vi "ROI_Setting_UI.vi"(8 "error in (no error)":errorcluster, 11 "Vision_Image":T1(plugin-control)) -> (0 "error out":errorcluster)   [LabVIEW 2019]
uses:
  Controls/ROI_List_Action.ctl
panel:
  in  "Exit":bool
  in  "RemoveROI":bool
  in  "CreateROI":bool
  in  "ROI List":i32[](listbox)
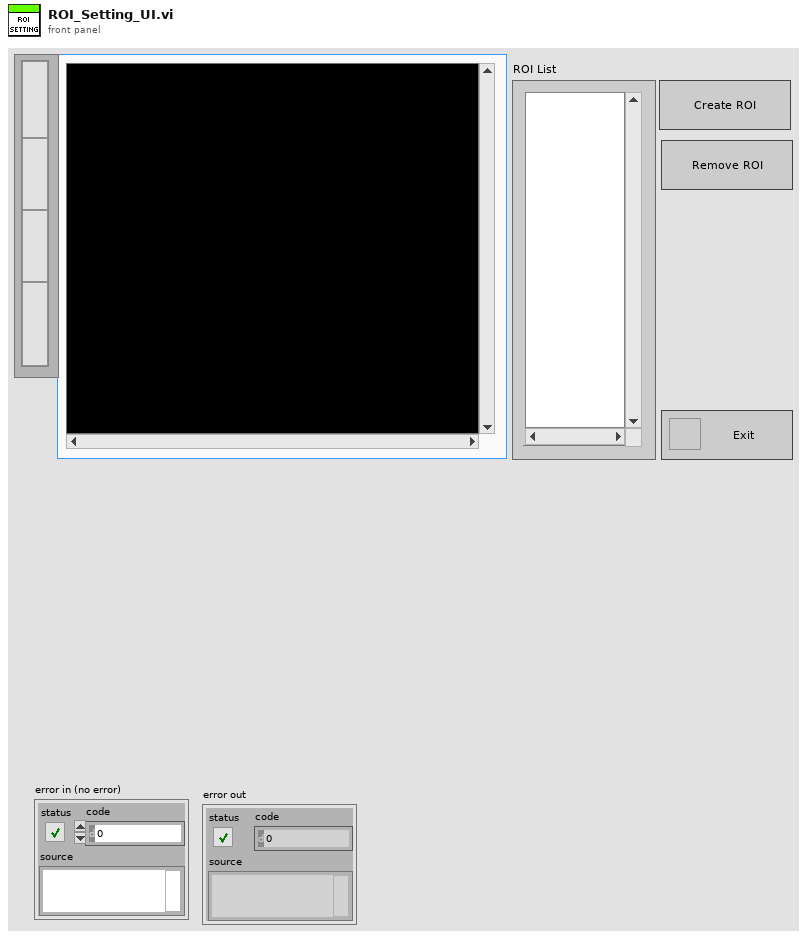
[diagram p1: front panel]
types:
  T1 = typedef "IMAQ Image.ctl" = refnum<image>
  T2 = typedef "ROI_List_Action.ctl" = enum16{"Init", "Add ROI", "Delete ROI", "Get All ROI", "Get Specific ROI", "Set Analysis Setting", "Set Process Setting", "Replace All Entries", "ROIEntryBackup", "ROIEntryBackupClear", "ROIEntryReturn"}
  T3 = cluster{"Global Rectangle":i32[], "Contours":cluster{"Contour Type":u32, "ROI Type":u32, "Points":i32[]}[]}
  T4 = cluster{"Contour Type":u32, "ROI Type":u32, "Points":i32[]}[]
  T5 = cluster{"Contour Type":u32, "ROI Type":u32, "Points":i32[]}
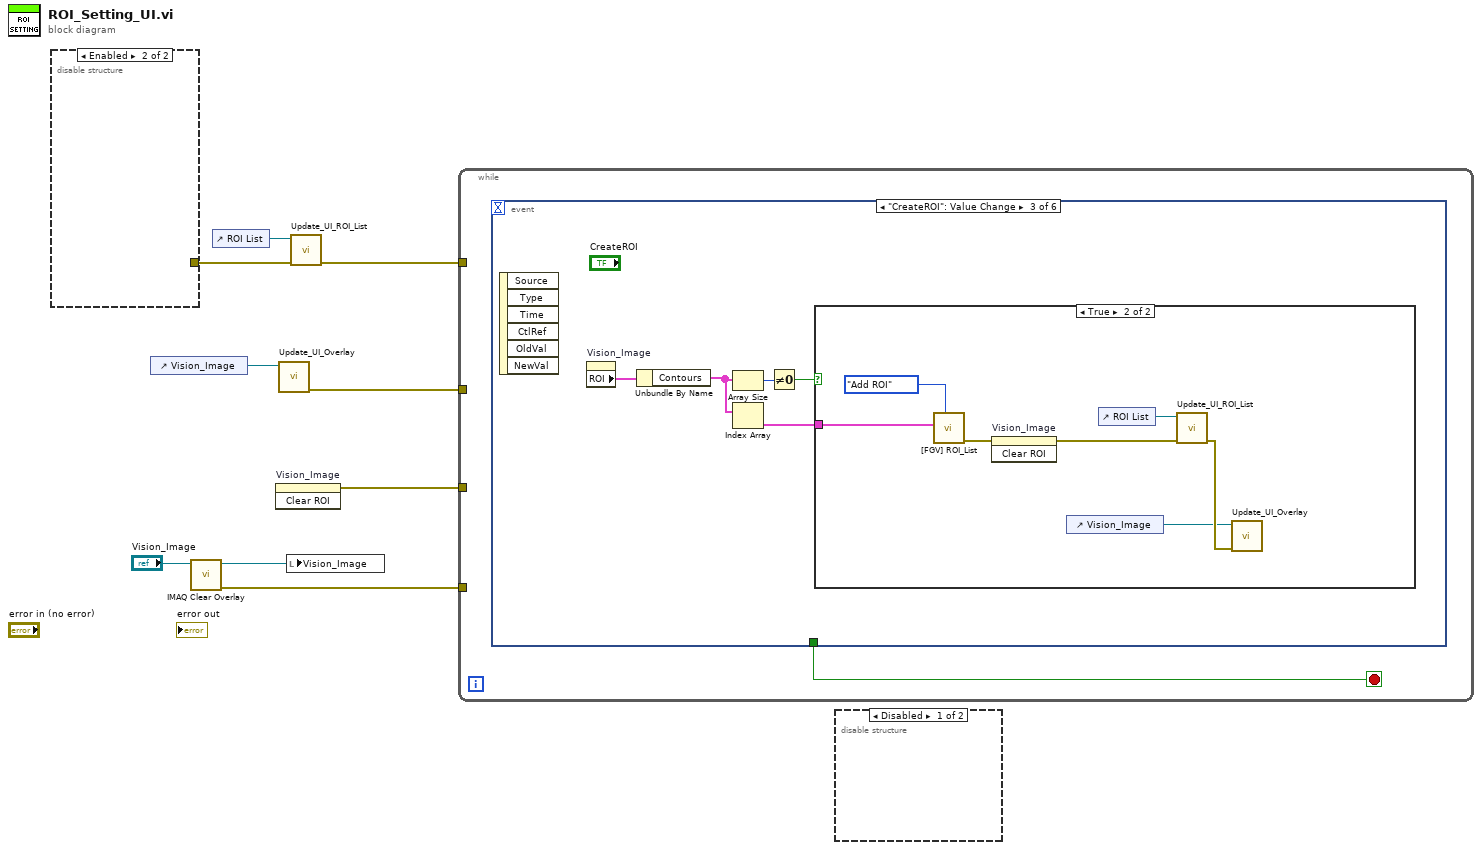
[diagram p0: block diagram]
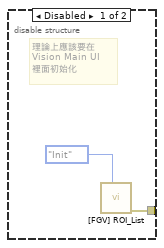
[diagram p3: hidden frame]
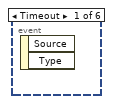
[diagram p4: hidden frame]
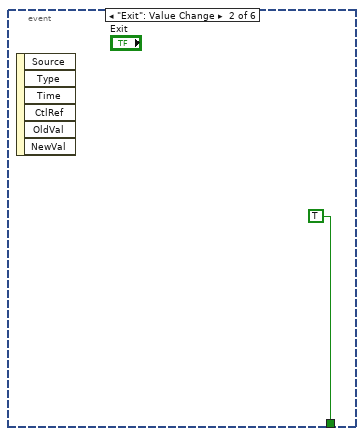
[diagram p5: hidden frame]
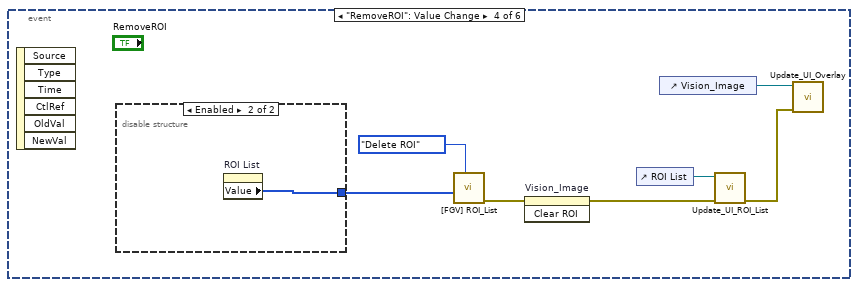
[diagram p7: hidden frame]
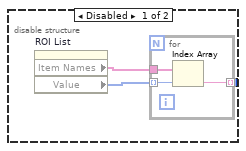
[diagram p8: hidden frame]
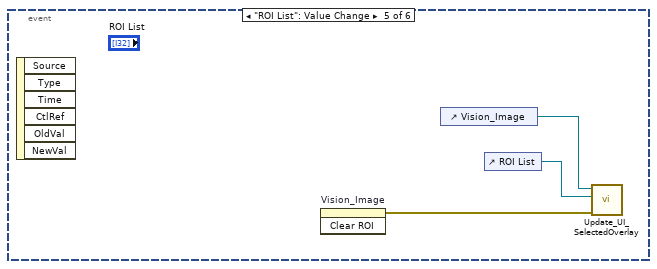
[diagram p9: hidden frame]
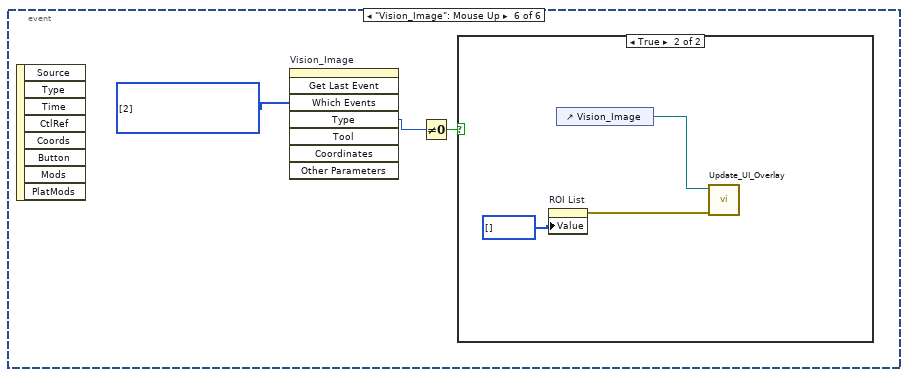
[diagram p10: hidden frame]
diagram:
  n1 = disable-structure shown="Enabled" {
    disable-tunnel: [w10 _] -> w7
    frame Disabled {
      # "理論上應該要在\nVision Main UI\n裡面初始化"
      n2 = call "[FGV] ROI_List.vi"("Action"=ROI_List_Action."Init") -> ("error out"=w10:errorcluster)  [unwired: 8 in, 2 out]
    }
    frame Enabled {
    }
  }
  n3 = control-ref of="Vision_Image"() -> (w2:refnum<vi>)
  n4 = call "IMAQ Clear Overlay"("Image"="Vision_Image") -> ("error out"=w3:errorcluster, "Image Out"=w4:T1)  [unwired: 9 in]
  n5 = control-ref of="ROI List"() -> (w8:refnum<vi>)
  n6 = invoke on="Vision_Image" class="ImageControl" method="Clear ROI"() -> (error out=w9:errorcluster)  [unwired: 3 in, 2 out]
  n7 = call "Update_UI_Overlay.vi"("Image Refnum"=w2) -> ("error out"=w1:errorcluster)  [unwired: 10 in]
  n8 = local write "Vision_Image"(w4) -> ()
  n9 = call "Update_UI_ROI_List.vi"("error in (no error)"=w7, "LstBox Refnum"=w8) -> ("error out"=w6:errorcluster)  [unwired: 9 in]
  n10 = while {
    tunnel: w9 -> [_]
    tunnel: w6 -> [_]
    tunnel: w3 -> [_]
    tunnel: w1 -> [_]
    stop <- w12 stop-if-true
    n11 = event shown="[2] \"CreateROI\": Value Change" {
      selector: _ -> [_ _ _ _ _ _]
      dyn-events: _ -> [_ _ _ _ _ _]
      timeout: _ -> [_ _ _ _ _ _]
      tunnel: [_ TRUE _ _ _ _] -> w12
      event Timeout {
        n12 = event-data() -> ()  [unwired: 1 in, 2 out]
      }
      event "Exit": Value Change {
        n13 = event-data() -> ()  [unwired: 1 in, 6 out]
      }
      event "CreateROI": Value Change {
        n14 = event-data() -> ()  [unwired: 1 in, 6 out]
        n15 = property on="Vision_Image" class="ImageControl"() -> ("ROI"=w18:T3)  [unwired: 2 in, 2 out]
        n16 = Unbundle By Name(w18) -> ("Contours"=w15:T4)
        n17 = Array Size(array=w15) -> (size(s)=w17:i32)
        n18 = Index Array(array=w15) -> (element=w14:T5)  [unwired: 1 in]
        n19 = Not Equal To 0?(x=w17) -> (x != 0?=w16:bool)
        n20 = case shown="True" w16 {
          tunnel: w14 -> [_ w24]
          frame False {
          }
          frame True {
            n21 = call "[FGV] ROI_List.vi"("Action"=ROI_List_Action."Add ROI", "ROI_To_Add"=w24) -> ("error out"=w23:errorcluster)  [unwired: 7 in, 2 out]
            n22 = invoke on="Vision_Image" class="ImageControl" method="Clear ROI"(error in=w23) -> (error out=w22:errorcluster)  [unwired: 2 in, 2 out]
            n23 = control-ref of="Vision_Image"() -> (w19:refnum<vi>)
            n24 = control-ref of="ROI List"() -> (w21:refnum<vi>)
            n25 = call "Update_UI_ROI_List.vi"("error in (no error)"=w22, "LstBox Refnum"=w21) -> ("error out"=w20:errorcluster)  [unwired: 9 in]
            n26 = call "Update_UI_Overlay.vi"("error in (no error)"=w20, "Image Refnum"=w19) -> ()  [unwired: 9 in, 1 out]
          }
        }
      }
      event "RemoveROI": Value Change {
        n27 = event-data() -> ()  [unwired: 1 in, 6 out]
        n28 = disable-structure shown="Enabled" {
          disable-tunnel: [w33 w39] -> w31
          frame Disabled {
            n29 = property on="ROI List" class="LstBox (strict)"() -> ("Item Names"=w35:string[], "Value"=w34:i32[])  [unwired: 2 in, 2 out]
            n30 = for {
              tunnel: w35 -> [w38]
              tunnel: w34 -> [w37] mode=indexing
              tunnel: [w36] -> w33 mode=indexing
              n31 = Index Array(array=w38, index=w37) -> (element=w36:string)
            }
          }
          frame Enabled {
            n32 = property on="ROI List" class="LstBox (strict)"() -> ("Value"=w39:i32[])  [unwired: 2 in, 2 out]
          }
        }
        n33 = call "[FGV] ROI_List.vi"("Action"=ROI_List_Action."Delete ROI", "ROIs_Index"=w31) -> ("error out"=w27:errorcluster)  [unwired: 7 in, 2 out]
        n34 = invoke on="Vision_Image" class="ImageControl" method="Clear ROI"(error in=w27) -> (error out=w26:errorcluster)  [unwired: 2 in, 2 out]
        n35 = control-ref of="ROI List"() -> (w30:refnum<vi>)
        n36 = control-ref of="Vision_Image"() -> (w29:refnum<vi>)
        n37 = call "Update_UI_ROI_List.vi"("error in (no error)"=w26, "LstBox Refnum"=w30) -> ("error out"=w28:errorcluster)  [unwired: 9 in]
        n38 = call "Update_UI_Overlay.vi"("error in (no error)"=w28, "Image Refnum"=w29) -> ()  [unwired: 9 in, 1 out]
      }
      event "ROI List": Value Change {
        n39 = event-data() -> ()  [unwired: 1 in, 6 out]
        n40 = invoke on="Vision_Image" class="ImageControl" method="Clear ROI"() -> (error out=w40:errorcluster)  [unwired: 3 in, 2 out]
        n41 = control-ref of="Vision_Image"() -> (w42:refnum<vi>)
        n42 = control-ref of="ROI List"() -> (w41:refnum<vi>)
        n43 = call "Update_UI_SelectedOverlay.vi"("error in (no error)"=w40, "LstBox Refnum"=w41, "Image Refnum"=w42) -> ()  [unwired: 8 in, 1 out]
      }
      event "Vision_Image": Mouse Up {
        w45 = i32[] [2] items=["No Event"=0, "Click Event"=1, "Draw Event"=2, "Size Event"=4, "Scroll Event"=5, "Double Click Event"=8] ("Which Events")
        n44 = event-data() -> ()  [unwired: 1 in, 8 out]
        n45 = invoke on="Vision_Image" class="ImageControl" method="Get Last Event"("Which Events"=w45) -> ("Type"=w44:i32)  [unwired: 7 in, 7 out]
        n46 = Not Equal To 0?(x=w44) -> (x != 0?=w43:bool)
        n47 = case shown="True" w43 {
          frame False {
          }
          frame True {
            n48 = property on="ROI List" class="LstBox (strict)"("Value"=i32[] [] ("ROI List")) -> (error out=w47:errorcluster)  [unwired: 2 in, 1 out]
            n49 = control-ref of="Vision_Image"() -> (w46:refnum<vi>)
            n50 = call "Update_UI_Overlay.vi"("error in (no error)"=w47, "Image Refnum"=w46) -> ()  [unwired: 9 in, 1 out]
          }
        }
      }
    }
  }
  n51 = disable-structure shown="Disabled" {
    frame Disabled {
    }
    frame Enabled {
    }
  }
